vi "disconnect.vi"(8 "error in (no error)":errorcluster, 11 "StimulatorAK101022TCP in":refnum<class "StimulatorAK101022TCP.lvclass">) -> (0 "error out":errorcluster, 3 "StimulatorAK101022TCP out":refnum<class "StimulatorAK101022TCP.lvclass">)   [LabVIEW 2010, in "StimulatorAK101022TCP.lvclass"]
uses:
  StimulatorAK101022TCP.lvclass
  StimulatorAK101022TCP.lvclass/StimulatorAK101022TCP.ctl
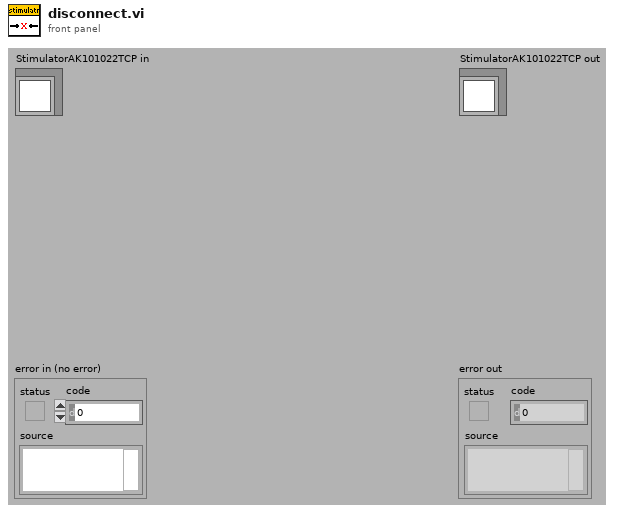
[diagram p1: front panel]
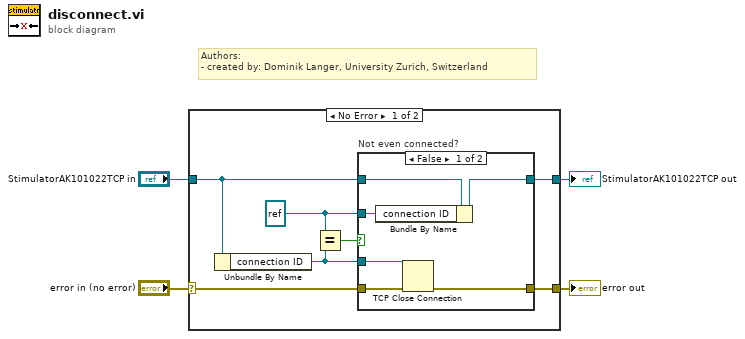
[diagram p0: block diagram]
diagram:
  # "Authors: \n- created by: Dominik Langer, University Zurich, Switzerland"
  n1 = case shown="No Error" "error in (no error)" {
    selector: "error in (no error)" -> [w9 w21]
    tunnel: [w8 w21] -> w3
    tunnel: [w10 w20] -> w1
    tunnel: "StimulatorAK101022TCP in" -> [w11 w20]
    frame No Error {
      w6 = refnum<k5> refnum ("connection ID")
      n2 = Unbundle By Name(w11) -> ("connection ID"=w7:refnum<k5>)
      n3 = Equal?(x=w6, y=w7) -> (x = y?=w5:bool)
      n4 = case "Not even connected?" shown="False" w5 {
        tunnel: w11 -> [w17 w19]
        tunnel: [w16 w19] -> w10
        tunnel: w9 -> [w15 w18]
        tunnel: [w14 w18] -> w8
        tunnel: w7 -> [w13 _]
        tunnel: w6 -> [w12 _]
        frame False {
          n5 = Bundle By Name(cluster=w17, "connection ID"=w12) -> (w16:refnum<class "StimulatorAK101022TCP.lvclass">)
          n6 = TCP Close Connection(connection ID=w13, error in (no error)=w15) -> (error out=w14:errorcluster)  [unwired: 1 in, 1 out]
        }
        frame True {
        }
      }
    }
    frame Error {
    }
  }
  "error out" <- w3
  "StimulatorAK101022TCP out" <- w1
